vi "Is Empty VArray.vi"(1 "Variant":variant) -> (0 "Empty VArray?":bool)   [LabVIEW 2020, in "openg_variant.lvlib"]
uses:
  openg_variant.lvlib
panel:
  # "EXPERIMENTAL"
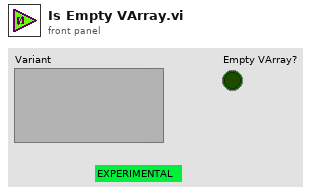
[diagram p1: front panel]
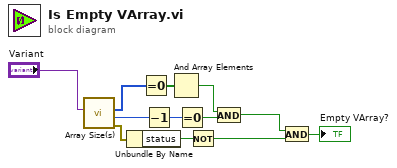
[diagram p0: block diagram]
diagram:
  n1 = call "Array Size(s).vi"("Array"="Variant") -> ("error out"=w11:errorcluster, "N dims"=w5:u32, "Size(s)"=w10:u32[])  [unwired: 8 in]
  n2 = Unbundle By Name(w11) -> ("status"=w8:bool)
  n3 = Equal To 0?(x=w10) -> (x = 0?=w9:bool[])
  n4 = Decrement(x=w5) -> (x-1=w4:u32)
  n5 = And Array Elements(Boolean array=w9) -> (logical AND=w2:bool)
  n6 = Equal To 0?(x=w4) -> (x = 0?=w3:bool)
  n7 = Not(x=w8) -> (.not. x?=w7:bool)
  n8 = And(x=w2, y=w3) -> (x .and. y?=w1:bool)
  n9 = And(x=w1, y=w7) -> (x .and. y?=→"Empty VArray?":bool)
